vi "S2C_FORNAX_Proc_CacheState.vi"(7 "Label":string, 8 "Error In":errorcluster, 11 "Data In":string) -> (0 "Error Out":errorcluster, 3 "Data Out":string)   [LabVIEW 2015]
uses:
  S2C_FORNAX_Proc_Globals.vi
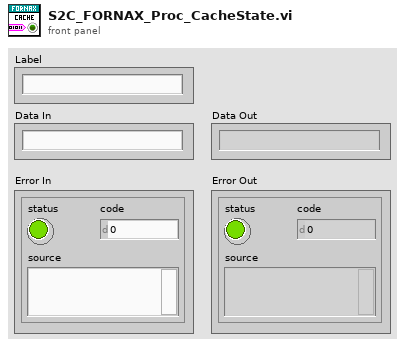
[diagram p1: front panel]
types:
  T1 = cluster{"VIP_Cmd":string, "VIP_RX":string, "VIP_Browse":bool, "VIP_Send":bool, "VIP_Clear":bool, "VipLogDepth":u32, "VIP_Auto":bool}
  T2 = cluster{"Partition":string, "Message":string, "M_destId":i32, "M_message":string, "M_Crc32":i32}
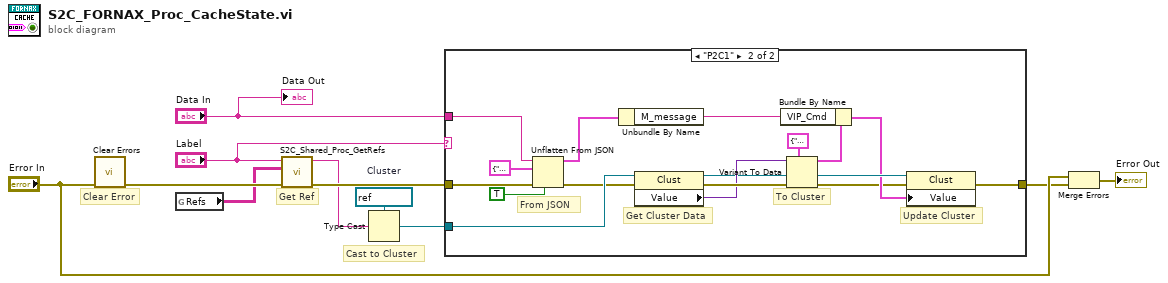
[diagram p0: block diagram]
diagram:
  w7 = refnum<vi> refnum  # Cluster
  # "Cast to Cluster"
  # "Get Ref"
  # "Clear Error"
  n1 = call <vilib>:"Clear Errors.vi"("error in (no error)"="Error In") -> ("error out"=w4:errorcluster)  [unwired: 5 in, 1 out]
  n2 = global read "S2C_FORNAX_Proc_Globals.vi" "Refs"() -> (w1:string[][])
  n3 = call "S2C_Shared_Proc_GetRefs.vi"("Error In"=w4, "Refs"=w1, "Label"="Label") -> ("Error Out"=w9:errorcluster, "Reference"=w6:string)  [unwired: 7 in]
  n4 = Type Cast(type=w7, x=w6) -> (*(type *) &x=w5:refnum<vi>)
  n5 = case shown="\"P2C1\"" "Label" {
    tunnel: w9 -> [w12 w19]
    tunnel: [w12 w22] -> w2
    tunnel: w5 -> [_ w25]
    tunnel: "Data In" -> [_ w18]
    frame "Other", Default {
    }
    frame "P2C1" {
      # "From JSON"
      # "Update Cluster"
      # "To Cluster"
      # "Get Cluster Data"
      n6 = Unflatten From JSON(JSON string=w18, type and defaults=T2 {"Partition"="", "Message"="", "M_destId"=0, "M_message"="", "M_Crc32"=0}, default null elements? (F)=TRUE, error in (no error)=w19) -> (value=w16:T2, error out=w14:errorcluster)  [unwired: 3 in]
      n7 = Unbundle By Name(w16) -> ("M_message"=w15:string)
      n8 = property class="Clust"(reference=w25, error in=w14) -> (reference out=w24:refnum<vi>, error out=w28:errorcluster, "Value"=w27:variant)
      n9 = Variant To Data(error in=w28, type=T1 {"VIP_Cmd"="boardid", "VIP_RX"="", "VIP_Browse"=FALSE, "VIP_Send"=FALSE, "VIP_Clear"=FALSE, "VipLogDepth"=50, "VIP_Auto"=TRUE} ("P2C1"), Variant=w27) -> (data=w26:T1, error out=w21:errorcluster)
      n10 = Bundle By Name(cluster=w26, "VIP_Cmd"=w15) -> (w23:T1)
      n11 = property class="Clust"(reference=w24, error in=w21, "Value"=w23) -> (error out=w22:errorcluster)  [unwired: 1 out]
    }
  }
  n12 = Merge Errors("Error In", w2) -> (→"Error Out":errorcluster)
  "Data Out" <- "Data In"
